vi "test.vi"() -> ()   [LabVIEW 2018]
uses:
  Socket/Socket.lvclass
  <vilib>/addons/zeromq/socket_type.ctl
  <vilib>/addons/zeromq/socket_options.ctl
  <vilib>/addons/zeromq/zeromq.lvlib
panel:
  in  "stop":bool
  out "received message 3":string
  out "received message 2":string
  out "received message":string
  out "error out":errorcluster
  in  "Socket in":refnum<class "Socket.lvclass">
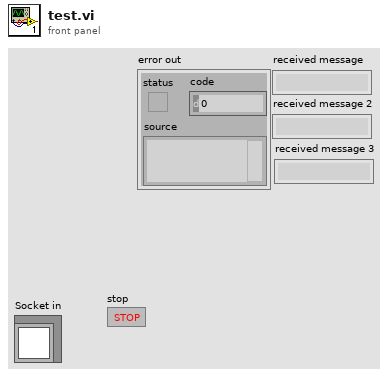
[diagram p1: front panel]
types:
  T1 = typedef "zeromq.lvlib/socket_type.ctl" = enum8{"ZMQ_PAIR", "ZMQ_PUB", "ZMQ_SUB", "ZMQ_REQ", "ZMQ_REP", "ZMQ_DEALER", "ZMQ_ROUTER", "ZMQ_PULL", "ZMQ_PUSH", "ZMQ_XPUB", "ZMQ_XSUB", "ZMQ_STREAM", "ZMQ_SERVER", "ZMQ_CLIENT", "ZMQ_RADIO", "ZMQ_DISH", "ZMQ_GATHER", "ZMQ_SCATTER", "ZMQ_DGRAM"}
  T2 = typedef "zeromq.lvlib/socket_options.ctl" = enum8{"NONE", "ZMQ_HWM", "<2>", "ZMQ_SWAP", "ZMQ_AFFINITY", "ZMQ_ROUTING_ID", "ZMQ_SUBSCRIBE", "ZMQ_UNSUBSCRIBE", "ZMQ_RATE", "ZMQ_RECOVERY_IVL", "ZMQ_MCAST_LOOP", "ZMQ_SNDBUF", "ZMQ_RCVBUF", "ZMQ_RCVMORE", "ZMQ_FD", "ZMQ_EVENTS", "ZMQ_TYPE", "ZMQ_LINGER", "ZMQ_RECONNECT_IVL", "ZMQ_BACKLOG", "ZMQ_RECOVERY_IVL_MSEC", "ZMQ_RECONNECT_IVL_MAX", "ZMQ_MAXMSGSIZE", "ZMQ_SNDHWM", "ZMQ_RCVHWM", "ZMQ_MULTICAST_HOPS", "<26>", "ZMQ_RCVTIMEO", "ZMQ_SNDTIMEO", "<29>", "<30>", "ZMQ_IPV4ONLY", "ZMQ_LAST_ENDPOINT", "ZMQ_ROUTER_MANDATORY", "ZMQ_TCP_KEEPALIVE", "ZMQ_TCP_KEEPALIVE_CNT", "ZMQ_TCP_KEEPALIVE_IDLE", "ZMQ_TCP_KEEPALIVE_INTVL", "ZMQ_TCP_ACCEPT_FILTER", "ZMQ_IMMEDIATE", "ZMQ_XPUB_VERBOSE", "ZMQ_ROUTER_RAW", "ZMQ_IPV6", "ZMQ_MECHANISM", "ZMQ_PLAIN_SERVER", "ZMQ_PLAIN_USERNAME", "ZMQ_PLAIN_PASSWORD", "ZMQ_CURVE_SERVER", "ZMQ_CURVE_PUBLICKEY", "ZMQ_CURVE_SECRETKEY", "ZMQ_CURVE_SERVERKEY", "ZMQ_PROBE_ROUTER", "ZMQ_REQ_CORRELATE", "ZMQ_REQ_RELAXED", "ZMQ_CONFLATE", "ZMQ_ZAP_DOMAIN", "ZMQ_ROUTER_HANDOVER", "ZMQ_TOS", "ZMQ_IPC_FILTER_PID", "ZMQ_IPC_FILTER_UID", "ZMQ_IPC_FILTER_GID", "ZMQ_CONNECT_ROUTING_ID", "ZMQ_GSSAPI_SERVER", "ZMQ_GSSAPI_PRINCIPAL", "ZMQ_GSSAPI_SERVICE_PRINCIPAL", "ZMQ_GSSAPI_PLAINTEXT", "ZMQ_HANDSHAKE_IVL", "<67>", "ZMQ_SOCKS_PROXY", "ZMQ_XPUB_NODROP", "ZMQ_BLOCKY", "ZMQ_XPUB_MANUAL", "ZMQ_XPUB_WELCOME_MSG", "ZMQ_STREAM_NOTIFY", "ZMQ_INVERT_MATCHING", "ZMQ_HEARTBEAT_IVL", "ZMQ_HEARTBEAT_TTL", "ZMQ_HEARTBEAT_TIMEOUT", "ZMQ_XPUB_VERBOSER", "ZMQ_CONNECT_TIMEOUT", "ZMQ_TCP_MAXRT", "ZMQ_THREAD_SAFE", "<82>", "<83>", "ZMQ_MULTICAST_MAXTPDU", "ZMQ_VMCI_BUFFER_SIZE", "ZMQ_VMCI_BUFFER_MIN_SIZE", "ZMQ_VMCI_BUFFER_MAX_SIZE", "ZMQ_VMCI_CONNECT_TIMEOUT", "ZMQ_USE_FD", "ZMQ_GSSAPI_PRINCIPAL_NAMETYPE", "ZMQ_GSSAPI_SERVICE_PRINCIPAL_NAMETYPE", "ZMQ_BINDTODEVICE", "ZMQ_ZAP_ENFORCE_DOMAIN", "ZMQ_LOOPBACK_FASTPATH", "ZMQ_METADATA", "ZMQ_MULTICAST_LOOP", "ZMQ_ROUTER_NOTIFY"}
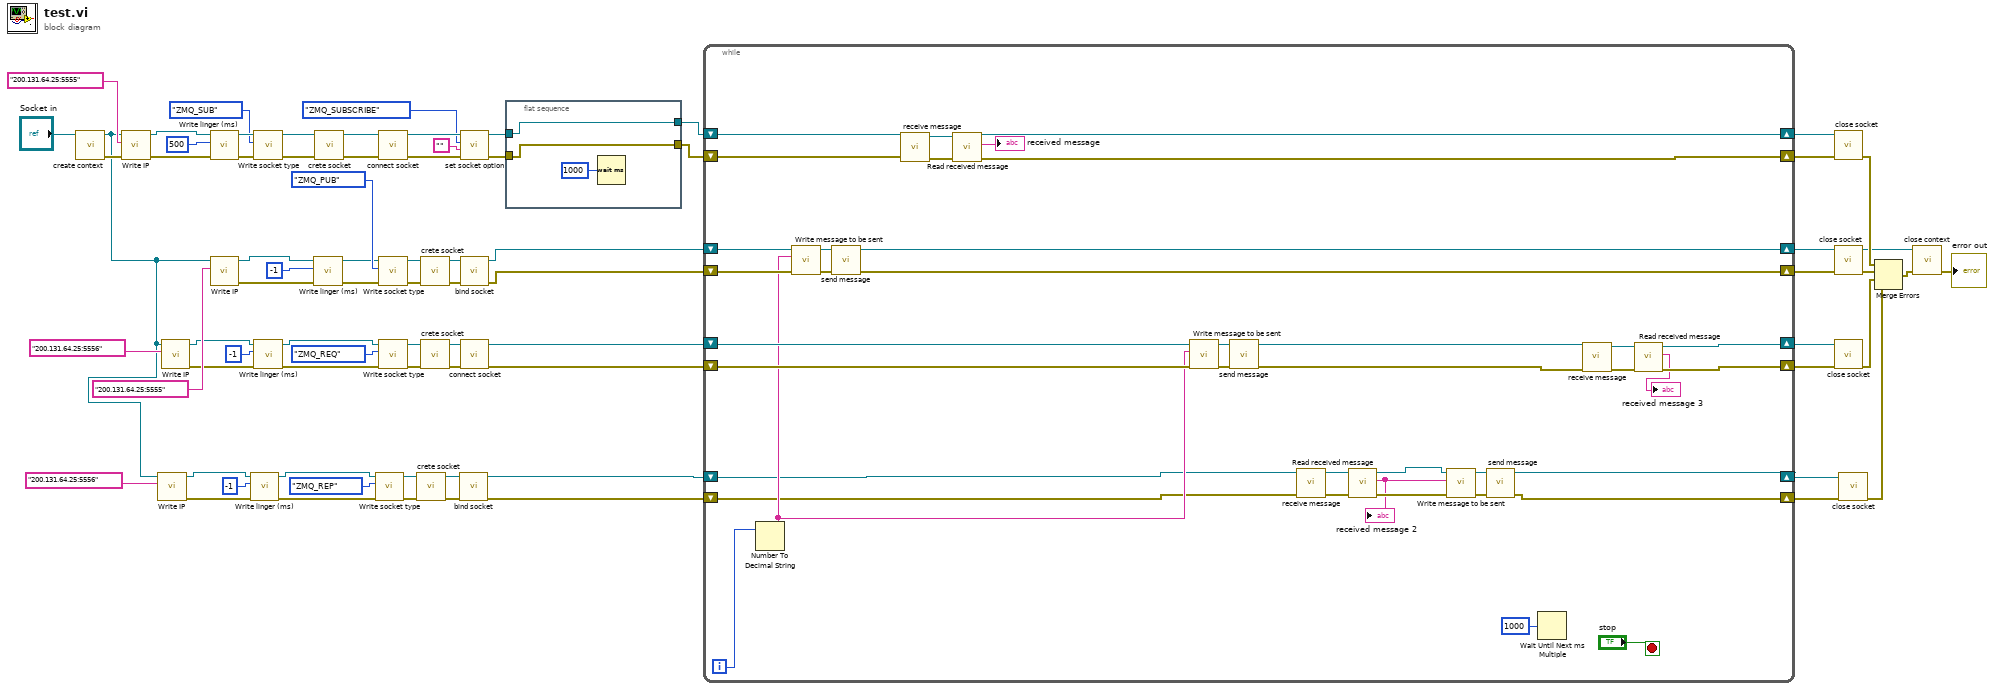
[diagram p0: block diagram]
diagram:
  n1 = call "create context.vi"("Socket in"="Socket in") -> ("error out"=w59:errorcluster, "Socket out"=w13:refnum<class "Socket.lvclass">)  [unwired: 9 in]
  n2 = call-dynamic "Write IP.vi"("error in (no error)"=w59, "IP"="200.131.64.25:5555", "Socket in"=w13) -> ("error out"=w71:errorcluster, "Socket out"=w74:refnum<class "Socket.lvclass">)  [unwired: 7 in]
  n3 = call-dynamic "Write IP.vi"("IP"="200.131.64.25:5556", "Socket in"=w13) -> ("error out"=w23:errorcluster, "Socket out"=w22:refnum<class "Socket.lvclass">)  [unwired: 8 in]
  n4 = call-dynamic "Write IP.vi"("IP"="200.131.64.25:5556", "Socket in"=w13) -> ("error out"=w34:errorcluster, "Socket out"=w36:refnum<class "Socket.lvclass">)  [unwired: 8 in]
  n5 = call-dynamic "Write linger (ms).vi"("error in (no error)"=w71, "linger (ms)"=500, "Socket in"=w74) -> ("error out"=w72:errorcluster, "Socket out"=w73:refnum<class "Socket.lvclass">)  [unwired: 7 in]
  n6 = call-dynamic "Write IP.vi"("IP"="200.131.64.25:5555", "Socket in"=w13) -> ("error out"=w53:errorcluster, "Socket out"=w50:refnum<class "Socket.lvclass">)  [unwired: 8 in]
  n7 = call-dynamic "Write linger (ms).vi"("error in (no error)"=w23, "linger (ms)"=-1, "Socket in"=w22) -> ("error out"=w24:errorcluster, "Socket out"=w21:refnum<class "Socket.lvclass">)  [unwired: 7 in]
  n8 = call-dynamic "Write socket type.vi"("error in (no error)"=w72, "Socket type"=socket_type."ZMQ_SUB", "Socket in"=w73) -> ("error out"=w60:errorcluster, "Socket out"=w61:refnum<class "Socket.lvclass">)  [unwired: 7 in]
  n9 = call-dynamic "Write linger (ms).vi"("error in (no error)"=w34, "linger (ms)"=-1, "Socket in"=w36) -> ("error out"=w33:errorcluster, "Socket out"=w37:refnum<class "Socket.lvclass">)  [unwired: 7 in]
  n10 = call-dynamic "Write linger (ms).vi"("error in (no error)"=w53, "linger (ms)"=-1, "Socket in"=w50) -> ("error out"=w52:errorcluster, "Socket out"=w51:refnum<class "Socket.lvclass">)  [unwired: 7 in]
  n11 = call "crete socket.vi"("error in (no error)"=w60, "Socket in"=w61) -> ("error out"=w75:errorcluster, "Socket out"=w76:refnum<class "Socket.lvclass">)  [unwired: 8 in]
  n12 = call-dynamic "Write socket type.vi"("error in (no error)"=w24, "Socket type"=socket_type."ZMQ_REP", "Socket in"=w21) -> ("error out"=w25:errorcluster, "Socket out"=w18:refnum<class "Socket.lvclass">)  [unwired: 7 in]
  n13 = call "connect socket.vi"("error in (no error)"=w75, "Socket in"=w76) -> ("error out"=w67:errorcluster, "Socket out"=w68:refnum<class "Socket.lvclass">)  [unwired: 8 in]
  n14 = call-dynamic "Write socket type.vi"("error in (no error)"=w52, "Socket type"=socket_type."ZMQ_PUB", "Socket in"=w51) -> ("error out"=w45:errorcluster, "Socket out"=w46:refnum<class "Socket.lvclass">)  [unwired: 7 in]
  n15 = call-dynamic "Write socket type.vi"("error in (no error)"=w33, "Socket type"=socket_type."ZMQ_REQ", "Socket in"=w37) -> ("error out"=w32:errorcluster, "Socket out"=w40:refnum<class "Socket.lvclass">)  [unwired: 7 in]
  n16 = call "crete socket.vi"("error in (no error)"=w25, "Socket in"=w18) -> ("error out"=w17:errorcluster, "Socket out"=w16:refnum<class "Socket.lvclass">)  [unwired: 8 in]
  n17 = call "crete socket.vi"("error in (no error)"=w45, "Socket in"=w46) -> ("error out"=w48:errorcluster, "Socket out"=w49:refnum<class "Socket.lvclass">)  [unwired: 8 in]
  n18 = call "crete socket.vi"("error in (no error)"=w32, "Socket in"=w40) -> ("error out"=w31:errorcluster, "Socket out"=w35:refnum<class "Socket.lvclass">)  [unwired: 8 in]
  n19 = call "bind socket.vi"("error in (no error)"=w17, "Socket in"=w16) -> ("error out"=w14:errorcluster, "Socket out"=w15:refnum<class "Socket.lvclass">)  [unwired: 8 in]
  n20 = call "set socket option.vi"("error in (no error)"=w67, "value"="", "option"=socket_options."ZMQ_SUBSCRIBE", "Socket2 in"=w68) -> ("error out"=w4:errorcluster, "Socket2 out"=w3:refnum<class "Socket.lvclass">)  [unwired: 6 in]
  n21 = call "bind socket.vi"("error in (no error)"=w48, "Socket in"=w49) -> ("error out"=w5:errorcluster, "Socket out"=w6:refnum<class "Socket.lvclass">)  [unwired: 8 in]
  n22 = call "connect socket.vi"("error in (no error)"=w31, "Socket in"=w35) -> ("error out"=w27:errorcluster, "Socket out"=w28:refnum<class "Socket.lvclass">)  [unwired: 8 in]
  n23 = flat-sequence {
    tunnel: w3 -> [w79]
    tunnel: [w79] -> w1
    tunnel: w4 -> [w78]
    tunnel: [w78] -> w2
    frame #0 {
      n24 = Wait (ms)(milliseconds to wait=u32 1000) -> ()  [unwired: 1 out]
    }
  }
  n25 = while {
    shift-right: [w118] -> w63
    shift-left: w1 -> [w97]
    shift-right: [w117] -> w62
    shift-left: w2 -> [w98]
    shift-right: [w116] -> w47
    shift-left: w6 -> [w115]
    shift-right: [w99] -> w7
    shift-left: w5 -> [w114]
    shift-right: [w111] -> w12
    shift-left: w28 -> [w113]
    shift-right: [w110] -> w11
    shift-left: w27 -> [w112]
    shift-right: [w109] -> w10
    shift-left: w15 -> [w103]
    shift-right: [w108] -> w8
    shift-left: w14 -> [w102]
    i -> [w106]
    stop <- "stop" stop-if-true
    n26 = Number To Decimal String(number=w106) -> (decimal integer string=w105:string)  [unwired: 1 in]
    n27 = call-dynamic "Write message to be sent.vi"("error in (no error)"=w114, "message to be sent"=w105, "Socket in"=w115) -> ("error out"=w96:errorcluster, "Socket out"=w95:refnum<class "Socket.lvclass">)  [unwired: 7 in]
    n28 = call "send message.vi"("error in (no error)"=w96, "Socket in"=w95) -> ("error out"=w99:errorcluster, "Socket out"=w116:refnum<class "Socket.lvclass">)  [unwired: 8 in]
    n29 = call-dynamic "receive message.vi"("error in (no error)"=w98, "Socket in"=w97) -> ("error out"=w93:errorcluster, "Socket out"=w92:refnum<class "Socket.lvclass">)  [unwired: 8 in]
    n30 = call-dynamic "Read received message.vi"("error in (no error)"=w93, "Socket in"=w92) -> ("error out"=w117:errorcluster, "received message"=→"received message":string, "Socket out"=w118:refnum<class "Socket.lvclass">)  [unwired: 7 in]
    n31 = call-dynamic "Write message to be sent.vi"("error in (no error)"=w112, "message to be sent"=w105, "Socket in"=w113) -> ("error out"=w91:errorcluster, "Socket out"=w90:refnum<class "Socket.lvclass">)  [unwired: 7 in]
    n32 = call "send message.vi"("error in (no error)"=w91, "Socket in"=w90) -> ("error out"=w100:errorcluster, "Socket out"=w101:refnum<class "Socket.lvclass">)  [unwired: 8 in]
    n33 = call-dynamic "receive message.vi"("error in (no error)"=w102, "Socket in"=w103) -> ("error out"=w88:errorcluster, "Socket out"=w89:refnum<class "Socket.lvclass">)  [unwired: 8 in]
    n34 = call-dynamic "Read received message.vi"("error in (no error)"=w88, "Socket in"=w89) -> ("error out"=w86:errorcluster, "received message"=w83:string, "Socket out"=w85:refnum<class "Socket.lvclass">)  [unwired: 7 in]
    "received message 2" <- w83
    n35 = call-dynamic "Write message to be sent.vi"("error in (no error)"=w86, "message to be sent"=w83, "Socket in"=w85) -> ("error out"=w87:errorcluster, "Socket out"=w84:refnum<class "Socket.lvclass">)  [unwired: 7 in]
    n36 = call "send message.vi"("error in (no error)"=w87, "Socket in"=w84) -> ("error out"=w108:errorcluster, "Socket out"=w109:refnum<class "Socket.lvclass">)  [unwired: 8 in]
    n37 = Wait Until Next ms Multiple(millisecond multiple=u32 1000) -> ()  [unwired: 1 out]
    n38 = call-dynamic "receive message.vi"("error in (no error)"=w100, "Socket in"=w101) -> ("error out"=w82:errorcluster, "Socket out"=w81:refnum<class "Socket.lvclass">)  [unwired: 8 in]
    n39 = call-dynamic "Read received message.vi"("error in (no error)"=w82, "Socket in"=w81) -> ("error out"=w110:errorcluster, "received message"=→"received message 3":string, "Socket out"=w111:refnum<class "Socket.lvclass">)  [unwired: 7 in]
  }
  n40 = call "close socket.vi"("error in (no error)"=w62, "Socket in"=w63) -> ("error out"=w42:errorcluster)  [unwired: 8 in, 1 out]
  n41 = call "close socket.vi"("error in (no error)"=w7, "Socket in"=w47) -> ("error out"=w44:errorcluster, "Socket out"=w41:refnum<class "Socket.lvclass">)  [unwired: 8 in]
  n42 = call "close socket.vi"("error in (no error)"=w11, "Socket in"=w12) -> ("error out"=w30:errorcluster)  [unwired: 8 in, 1 out]
  n43 = call "close socket.vi"("error in (no error)"=w8, "Socket in"=w10) -> ("error out"=w9:errorcluster)  [unwired: 8 in, 1 out]
  n44 = Merge Errors(w42, w44, w30, w9) -> (w43:errorcluster)
  n45 = call-dynamic "close context.vi"("error in (no error)"=w43, "Socket in"=w41) -> ("error out"=→"error out":errorcluster)  [unwired: 8 in, 1 out]
